vi "pickDefensiveTeam.vi"(0 "DefensiveTeam in":refnum<class "Ally.lvclass">, 1 "BallRef":refnum<class "Ball.lvclass">, 5 "KeeperTeam":refnum<class "Ally.lvclass">, 7 "OffensiveTeam":refnum<class "Ally.lvclass">, 9 "RobotRef in":refnum<class "Robot.lvclass">[](array[class]), 11 "error in (no error)":errorcluster, 12 "number_of_robots":i32) -> (4 "DefensiveTeam out":refnum<class "Ally.lvclass">, 8 "RobotRef":refnum<class "Robot.lvclass">[](array[class]), 15 "error out":errorcluster)   [LabVIEW 2023, in "Ally.lvclass"]
uses:
  Ally.lvclass
  Robot_class/Robot.lvclass
  Ball_class/Ball.lvclass
  Team_class/Team.lvclass/Team.ctl
  Utilities_class/Utilities.lvclass
  Robot_class/Robot.lvclass/Robot.ctl
  Robot_class/Read id.vi
  Team_class/Write RobotRef.vi
  Team_class/Read RobotRef.vi
  Team_class/Read DefensivePlay.vi
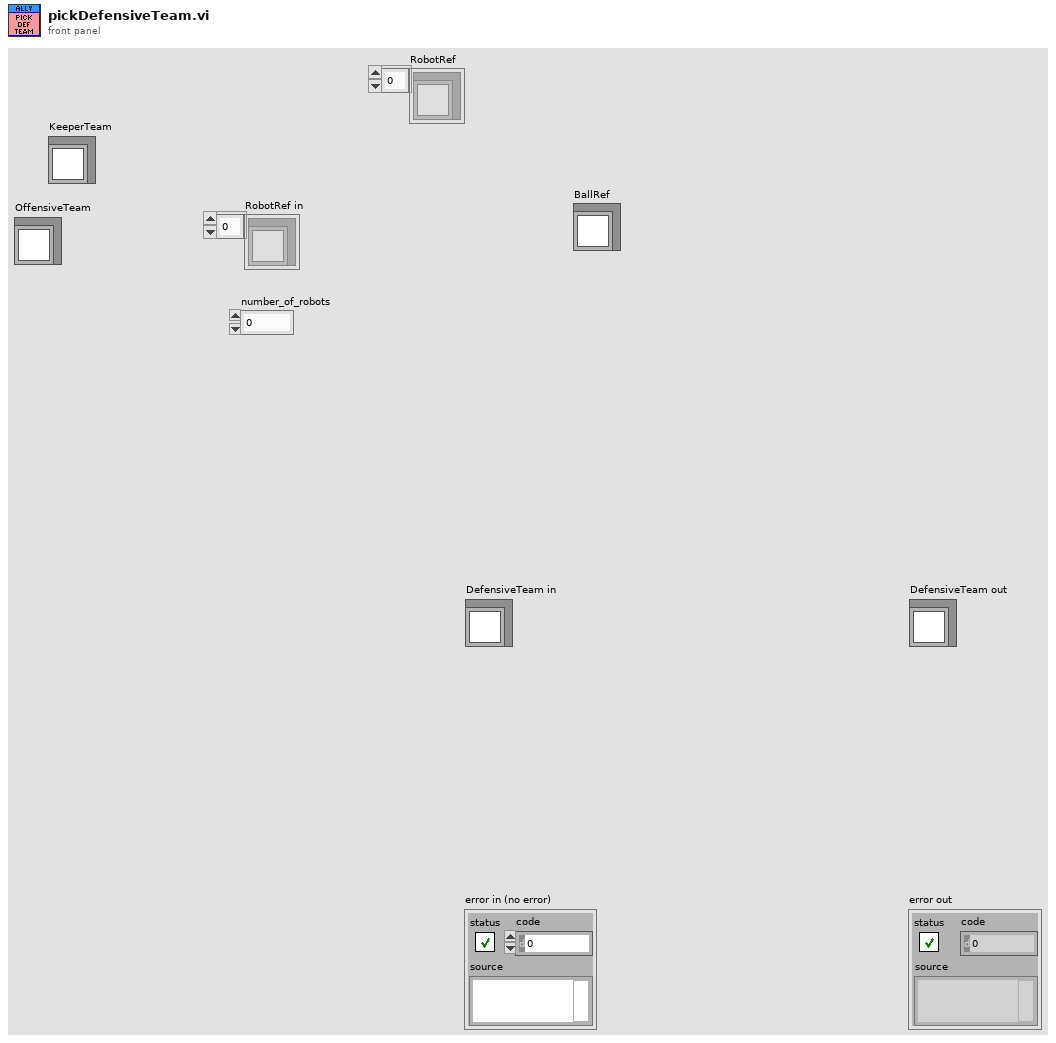
[diagram p1: front panel]
types:
  T1 = typedef "DefensivePlay.ctl" = enum16{"NormalDefensiveWithDuelist", "NormalDefensive", "TestPlay", "Halt", "Timeout", "PenaltyEnemy", "PenaltyAlly"}
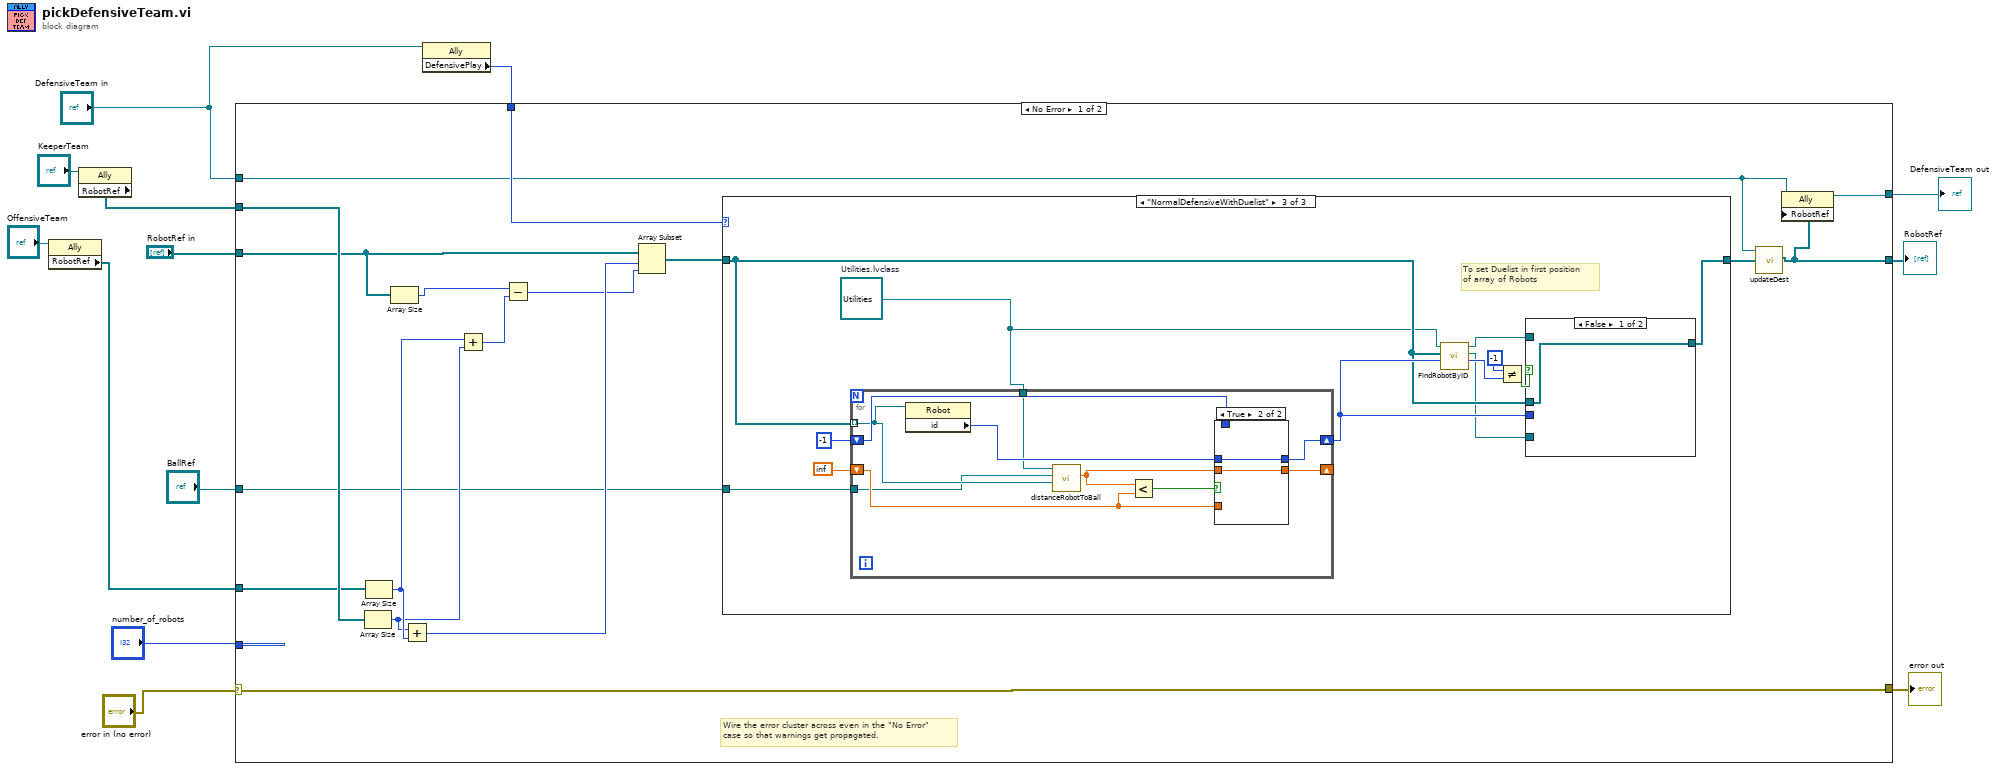
[diagram p0: block diagram]
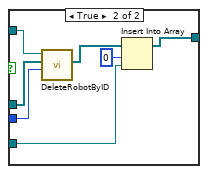
[diagram p4: hidden frame]
diagram:
  n1 = property class="Ally"(reference="OffensiveTeam") -> ("RobotRef"=w4:refnum<class "Robot.lvclass">[])  [unwired: 1 in, 2 out]
  n2 = property class="Ally"(reference="KeeperTeam") -> ("RobotRef"=w10:refnum<class "Robot.lvclass">[])  [unwired: 1 in, 2 out]
  n3 = property class="Ally"(reference="DefensiveTeam in") -> ("DefensivePlay"=w2:T1)  [unwired: 1 in, 2 out]
  n4 = case shown="No Error" "error in (no error)" {
    selector: "error in (no error)" -> [w30 w68]
    tunnel: [w30 w68] -> w6
    tunnel: [w29 w67] -> w7
    tunnel: "DefensiveTeam in" -> [w15 w67]
    tunnel: "RobotRef in" -> [w20 _]
    tunnel: "number_of_robots" -> [_ _]
    tunnel: w10 -> [w28 _]
    tunnel: [w16 _] -> w9
    tunnel: w4 -> [w27 _]
    tunnel: w2 -> [w25 _]
    tunnel: "BallRef" -> [w14 _]
    frame No Error {
      # "Wire the error cluster across even in the \"No Error\"\ncase so that warnings get propagated."
      n5 = Array Size(array=w28) -> (size(s)=w22:i32)
      n6 = Array Size(array=w27) -> (size(s)=w23:i32)
      n7 = Array Size(array=w20) -> (size(s)=w19:i32)
      n8 = Add(x=w22, y=w23) -> (x+y=w26:i32)
      n9 = Add(x=w23, y=w22) -> (x+y=w21:i32)
      n10 = Subtract(x=w19, y=w21) -> (x-y=w18:i32)
      n11 = Array Subset(array=w20, index=w26, length=w18) -> (w24:refnum<class "Robot.lvclass">[])
      n12 = case shown="\"NormalDefensiveWithDuelist\"" w25 {
        tunnel: [w31 w32 w40] -> w17
        tunnel: w24 -> [w31 w32 w39]
        tunnel: w14 -> [_ _ w33]
        frame "TestPlay" {
          # "Aqui entra a lógica para\nreeordenar o team de acordo \ncom quem deve assumir cada\nrole"
        }
        frame "NormalDefensive", Default {
        }
        frame "NormalDefensiveWithDuelist" {
          w38 = refnum<class "Utilities.lvclass"> refnum  # Utilities.lvclass
          # "To set Duelist in first position\nof array of Robots"
          n13 = for {
            tunnel: w39 -> [w54] mode=indexing
            shift-right: [w61] -> w43
            shift-left: -1 ("id") -> [w58]
            shift-right: [w59] -> _
            shift-left: inf -> [w57]
            tunnel: w38 -> [w56]
            tunnel: w33 -> [w53]
            n14 = property class="Robot"(reference=w54) -> ("id"=w60:i32)  [unwired: 1 in, 2 out]
            n15 = call "distanceRobotToBall.vi"("Robot"=w54, "Ball"=w53, "Utilities in"=w56) -> ("Distance Robot To Ball"=w55:dbl)  [unwired: 6 in, 2 out]
            n16 = Less?(x=w55, y=w57) -> (x < y?=w62:bool)
            n17 = case shown="True" w62 {
              tunnel: [w64 w66] -> w61
              tunnel: w60 -> [_ w66]
              tunnel: [w63 w65] -> w59
              tunnel: w55 -> [_ w65]
              tunnel: w58 -> [w64 _]
              tunnel: w57 -> [w63 _]
              frame False {
              }
              frame True {
              }
            }
          }
          n18 = call-dynamic "FindRobotByID.vi"("id"=w43, "RobotRef"=w39, "Utilities in"=w38) -> ("index"=w37:i32, "Robot"=w34:refnum<class "Robot.lvclass">, "Utilities out"=w42:refnum<class "Utilities.lvclass">)  [unwired: 5 in, 1 out]
          n19 = Not Equal?(x=-1, y=w37) -> (x != y?=w35:bool)
          n20 = case shown="False" w35 {
            tunnel: w43 -> [_ w50]
            tunnel: w42 -> [_ w52]
            tunnel: [w45 w46] -> w40
            tunnel: w39 -> [w45 w51]
            tunnel: w34 -> [_ w48]
            frame False {
            }
            frame True {
              n21 = call-dynamic "DeleteRobotByID.vi"("id"=w50, "RobotRef"=w51, "Utilities in"=w52) -> ("RobotRef out"=w49:refnum<class "Robot.lvclass">[])  [unwired: 6 in, 2 out]
              n22 = Insert Into Array(array=w49, index=0, new element=w48) -> (w46:refnum<class "Robot.lvclass">[])
            }
          }
        }
      }
      n23 = call "updateDest.vi"("NewAllyRobots"=w17, "LastAlly"=w15) -> ("NewAllyRobotsUpdated"=w16:refnum<class "Robot.lvclass">[])  [unwired: 7 in, 2 out]
      n24 = property class="Ally"(reference=w15, "RobotRef"=w16) -> (reference out=w29:refnum<class "Ally.lvclass">)  [unwired: 1 in, 1 out]
    }
    frame Error {
    }
  }
  "error out" <- w6
  "DefensiveTeam out" <- w7
  "RobotRef" <- w9
